vi "Auto Match.vi"() -> ()   [LabVIEW 2010]
doc: "This VI is the solution to an exercise in the LabVIEW Core I course.\n\nIt is used to demonstrate passing data out of a while loop through a tunnel. This VI generates random numbers until the generated number matches a specified value. The loop count terminal keeps track of the number of iterations before a match occurs."
panel:
  in  "Number to Match":dbl=50.0 min=0.0 max=1000.0 step=1.0
  out "# of iterations":i32
  out "Current Number":dbl
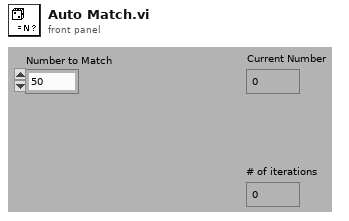
[diagram p1: front panel]
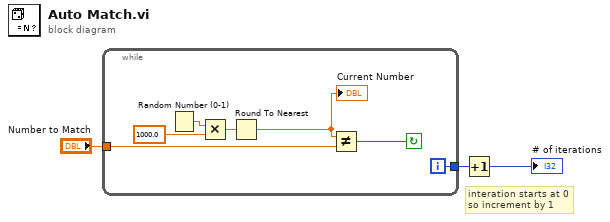
[diagram p0: block diagram]
diagram:
  # "interation starts at 0 so increment by 1"
  n1 = while {
    tunnel: [w5] -> w3
    tunnel: "Number to Match" -> [w4]
    i -> [w5]
    stop <- w6 continue-if-true
    n2 = Random Number (0-1)() -> (number: 0 to 1=w7:dbl)
    n3 = Multiply(x=w7, y=1000.0) -> (x*y=w9:dbl)
    n4 = Round To Nearest(number=w9) -> (nearest integer value=w10:dbl)
    "Current Number" <- w10
    n5 = Not Equal?(x=w10, y=w4) -> (x != y?=w6:bool)
  }
  n6 = Increment(x=w3) -> (x+1=→"# of iterations":i32)
